vi "exercícios2.vi"() -> ()   [LabVIEW 2018]
panel:
  out "Boolean 4":bool
  out "Boolean 3":bool
  in  "Boolean 2":bool
  out "Numeric 3":dbl
  out "Meter":sgl(knob) scale=0.0..10.0
  in  "Knob":sgl(knob) scale=0.0..10.0
  out "Tank":dbl(slide) scale=0.0..10.0
  in  "Slide":dbl(slide) scale=0.0..10.0
  out "String":string
  out "Boolean":bool=TRUE
  out "Numeric 2":dbl
  out "Numeric":i32
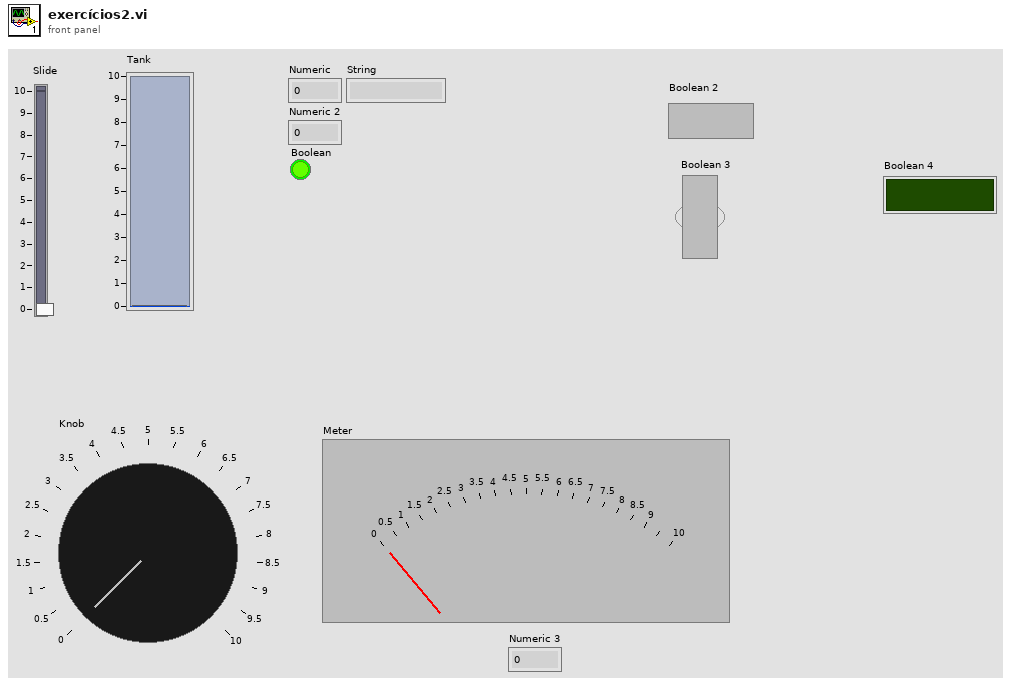
[diagram p1: front panel]
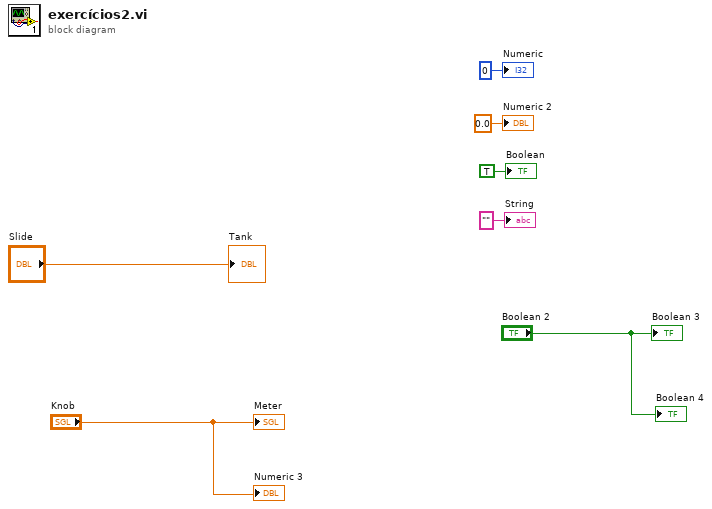
[diagram p0: block diagram]
diagram:
  "Numeric" <- 0
  "Numeric 2" <- 0.0
  "Boolean" <- TRUE
  "String" <- ""
  "Tank" <- "Slide"
  "Meter" <- "Knob"
  "Numeric 3" <- "Knob"
  "Boolean 3" <- "Boolean 2"
  "Boolean 4" <- "Boolean 2"
